vi "Reanimate.vi"(8 "Error In":errorcluster, 11 "Selection List[]":refnum<vi>[](array[refnum])) -> (0 "Error Out":errorcluster, 3 "Change Made?":bool)   [LabVIEW 2017, in "Eulogy.lvlib"]
doc: "Creates zombie code because once dead code is now alive (undead). Changes a grave site (Diagram Disable structure) to the Corpse frame (legacy code) and enables it. The \"Corpse\" label is replaced with a \"Zombie\" label and a timestamp of when the legacy code was re-enabled. In other words, infect the corpse with a zombie virus to revive it."
uses:
  Eulogy.lvlib
  Typedefs/Bookmarks.ctl
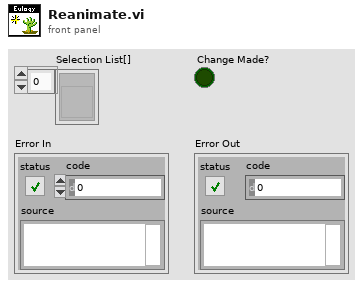
[diagram p1: front panel]
types:
  T1 = typedef "Eulogy.lvlib/Bookmarks.ctl" = enum16{"RIP", "Zombie"}
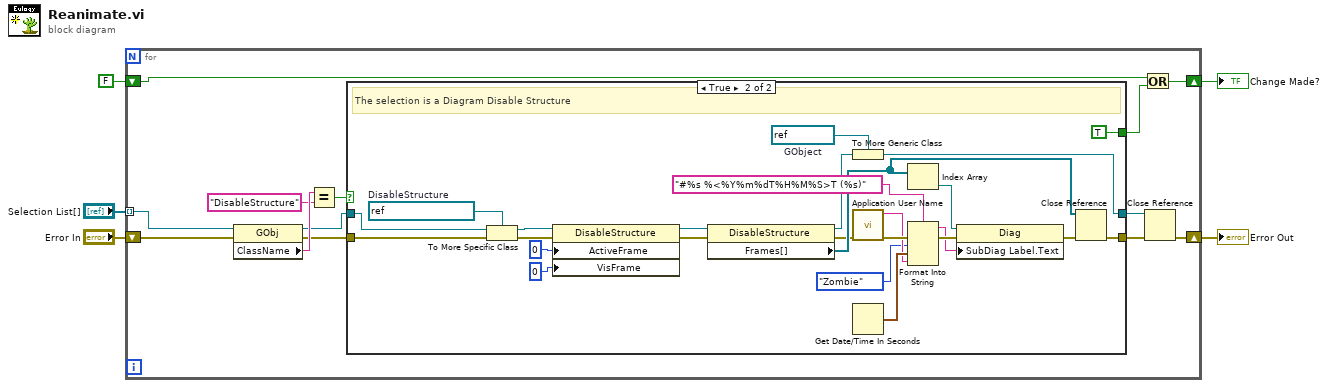
[diagram p0: block diagram]
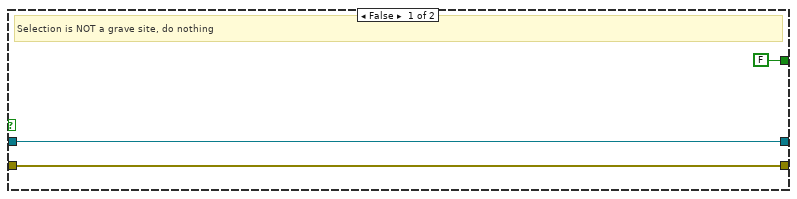
[diagram p2: hidden frame]
diagram:
  n1 = for {
    shift-right: [w6] -> w5
    shift-left: "Error In" -> [w18]
    tunnel: "Selection List[]" -> [w12] mode=indexing
    shift-right: [w9] -> w3
    shift-left: FALSE -> [w11]
    n2 = property class="GObj"(reference=w12, error in=w18) -> (reference out=w14:refnum<vi>, error out=w13:errorcluster, "ClassName"=w17:string)
    n3 = Equal?(x=w17, y="DisableStructure") -> (x = y?=w15:bool)
    n4 = case shown="True" w15 {
      tunnel: w14 -> [w20 w45]
      tunnel: w13 -> [w19 w44]
      tunnel: [FALSE ("y") TRUE ("y")] -> w10
      tunnel: [w19 w33] -> w8
      tunnel: [w20 w31] -> w7
      frame False {
        # "Selection is NOT a grave site, do nothing"
      }
      frame True {
        w30 = refnum<vi> refnum  # GObject
        w46 = refnum<vi> refnum  # DisableStructure
        # "The selection is a Diagram Disable Structure"
        n5 = To More Specific Class(target class=w46, reference=w45, error in=w44) -> (specific class reference=w42:refnum<vi>, error out=w43:errorcluster)
        n6 = property class="DisableStructure"(reference=w42, error in=w43, "ActiveFrame"=i16 0 ("Active Frame"), "VisFrame"=u32 0 ("Visible Frame")) -> (reference out=w39:refnum<vi>, error out=w38:errorcluster)
        n7 = property class="DisableStructure"(reference=w39, error in=w38) -> (reference out=w32:refnum<vi>, error out=w27:errorcluster, "Frames[]"=w35:refnum<vi>[])
        n8 = To More Generic Class(target class=w30, reference=w32) -> (generic class reference=w31:refnum<vi>)
        n9 = call "Application User Name.vi"("Error In"=w27) -> ("Error Out"=w26:errorcluster, "User Name"=w23:string)  [unwired: 9 in]
        n10 = Get Date/Time In Seconds() -> (seconds since 1Jan1904=w24:timestamp)
        n11 = Index Array(array=w35) -> (element=w37:refnum<vi>)  [unwired: 1 in]
        n12 = Format Into String(format string="#%s %<%Y%m%dT%H%M%S>T (%s)" ("time format string (%c)"), error in=w26, Bookmarks."Zombie" ("Bookmark"), w24, w23) -> (resulting string=w25:string, error out=w29:errorcluster)  [unwired: 1 in]
        n13 = property class="Diag"(reference=w37, error in=w29, "SubDiag Label.Text"=w25) -> (error out=w36:errorcluster)  [unwired: 1 out]
        n14 = Close Reference(reference=w35, error in (no error)=w36) -> (error out=w33:errorcluster)
      }
    }
    n15 = Or(x=w11, y=w10) -> (x .or. y?=w9:bool)
    n16 = Close Reference(reference=w7, error in (no error)=w8) -> (error out=w6:errorcluster)
  }
  "Error Out" <- w5
  "Change Made?" <- w3
